vi "Get_WheelVelocity.vi"(8 "error in":errorcluster, 11 "MG17Motor in":refnum<k7>) -> (0 "error out":errorcluster, 3 "pfWheelVel":sgl)   [LabVIEW 2021]
doc: "André Romero - 2023\nandretec@ifsc.usp.br\nIFSC - USP"
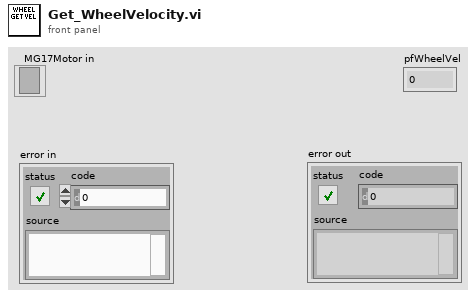
[diagram p1: front panel]
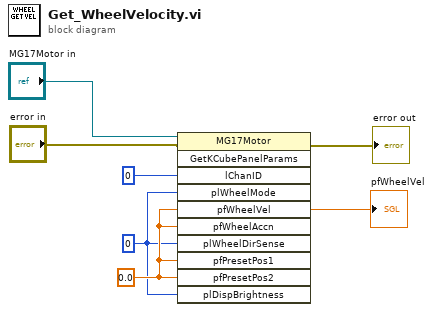
[diagram p0: block diagram]
diagram:
  w3 = 0 ("plWheelMode")
  w4 = sgl 0.0 ("pfPresetPos2")
  n1 = invoke class="MG17Motor" method="GetKCubePanelParams"(reference="MG17Motor in", error in="error in", "lChanID"=0, "plWheelMode"=w3, "pfWheelVel"=w4, "pfWheelAccn"=w4, "plWheelDirSense"=w3, "pfPresetPos1"=w4, "pfPresetPos2"=w4, "plDispBrightness"=w3) -> (error out=→"error out":errorcluster, "pfWheelVel"=→"pfWheelVel":sgl)  [unwired: 1 in, 9 out]
